vi "Trigger.vi"(8 "error in (no error)":errorcluster, 11 "VISA resource name":refnum<visa-resource-name>) -> (0 "error out":errorcluster, 3 "VISA resource name out":refnum<visa-resource-name>)   [LabVIEW 2014, in "LCR Meter.lvlib"]
doc: "Causes the trigger to execute a measurement or a sweep measurement, regardless of the trigger state.\n\n<B>Note</B>\nONLY used in BUS trigger mode."
uses:
  <instrlib>/LCR Meter/Examples/LCR Meter Acquire Single_1 Folder/LCR Meter.lvlib
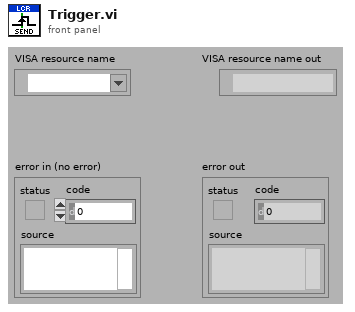
[diagram p1: front panel]
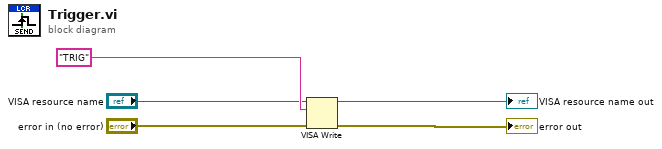
[diagram p0: block diagram]
diagram:
  n1 = VISA Write(VISA resource name="VISA resource name", write buffer="TRIG", error in (no error)="error in (no error)") -> (VISA resource name out=→"VISA resource name out":refnum<visa-resource-name>, error out=→"error out":errorcluster)  [unwired: 1 out]
